vi "Get Array Element at Index.vi"   [LabVIEW 2015, in "YAML Parser.lvclass"]
uses:
  YAML Parser.lvclass
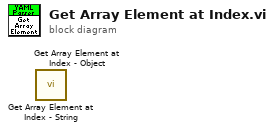
[diagram p0: block diagram]
diagram:
  n1 = call "Get Array Element at Index - String.vi"() -> ()  [unwired: 8 in, 4 out]
  n2 = call "Get Array Element at Index - Object.vi"() -> ()  [unwired: 8 in, 4 out]
